vi "Open File or Folder or EXE.vi"(8 "error in (no error)":errorcluster, 11 "Path":path) -> (0 "error out":errorcluster)   [LabVIEW 2016, in "SLL File IO.lvlib"]
doc: "Opens a File or Folder or EXE depending on the path specified."
uses:
  SLL File IO.lvlib
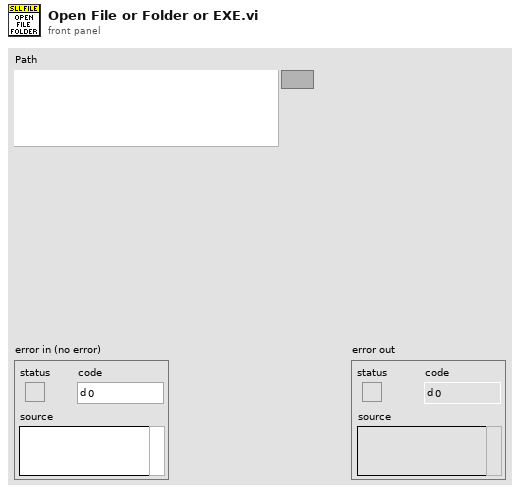
[diagram p1: front panel]
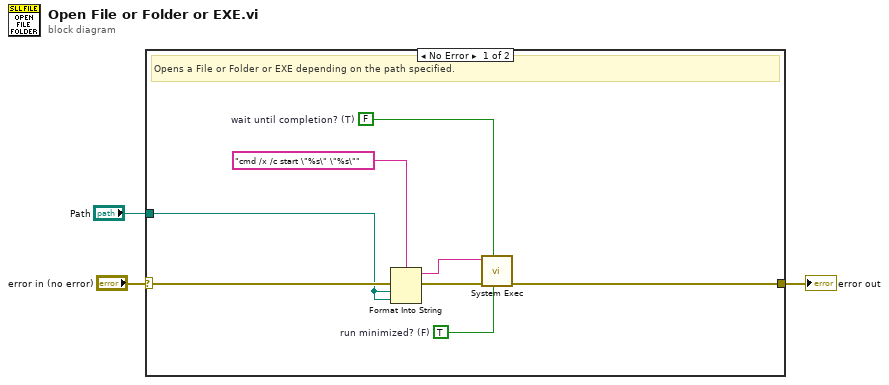
[diagram p0: block diagram]
diagram:
  n1 = case shown="No Error" "error in (no error)" {
    selector: "error in (no error)" -> [w11 w12]
    tunnel: [w10 w12] -> w2
    tunnel: "Path" -> [w4 _]
    frame No Error {
      w8 = TRUE  # run minimized? (F)
      w9 = FALSE  # wait until completion? (T)
      # "Opens a File or Folder or EXE depending on the path specified."
      n2 = Format Into String(format string="cmd /x /c start \"%s\" \"%s\"", error in=w11, w4, w4) -> (resulting string=w5:string, error out=w7:errorcluster)  [unwired: 1 in]
      n3 = call <vilib>:"System Exec.vi"("run minimized? (F)"=w8, "wait until completion? (T)"=w9, "error in (no error)"=w7, "command line"=w5) -> ("error out"=w10:errorcluster)  [unwired: 4 in, 3 out]
    }
    frame Error {
    }
  }
  "error out" <- w2
